vi "Update Support Build Specs and Build.vi"(7 "support build specs":T1, 8 "error in":errorcluster, 9 "CD support lvproj name":string, 10 "CD name":string, 11 "custom device path":path) -> (0 "error out":errorcluster, 3 "custom device path out":path)   [LabVIEW 2020, in "Template Tool.lvlib"]
uses:
  Template Tool.lvlib
  Project Build Specs.ctl
  <vilib>/AppBuilder/AB_API/PPL/NI_AB_API_PPL.lvclass
  <vilib>/AppBuilder/AB_API/SDIST/NI_AB_API_SDIST.lvclass
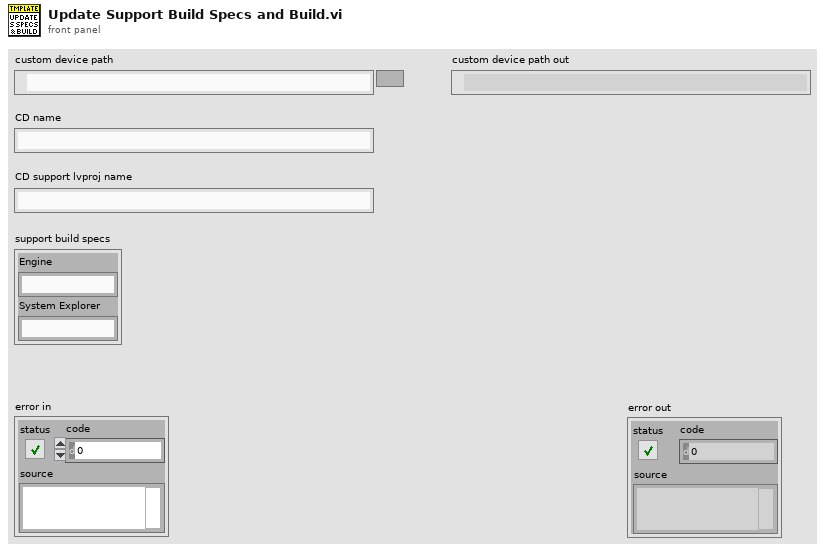
[diagram p1: front panel]
types:
  T1 = typedef "Template Tool.lvlib/Project Build Specs.ctl" = cluster{"Engine":string, "System Explorer":string}
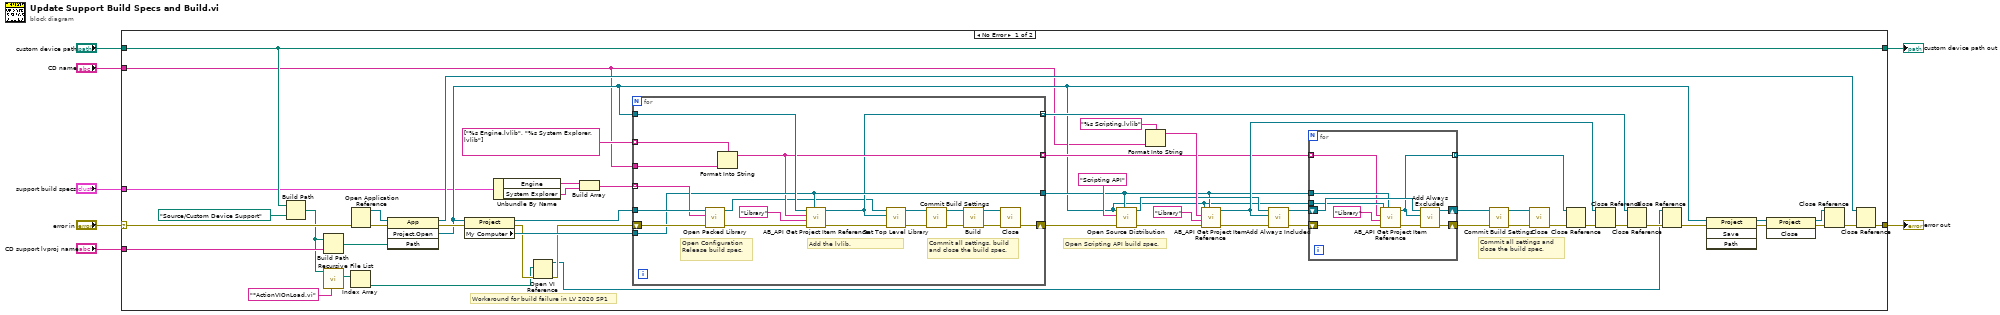
[diagram p0: block diagram]
diagram:
  n1 = case shown="No Error" "error in" {
    selector: "error in" -> [w61 w94]
    tunnel: "custom device path" -> [w53 w93]
    tunnel: [w54 w94] -> w7
    tunnel: [w53 w93] -> w4
    tunnel: "CD support lvproj name" -> [w22 _]
    tunnel: "CD name" -> [w21 _]
    tunnel: "support build specs" -> [w11 _]
    frame No Error {
      # "Workaround for build failure in LV 2020 SP1"
      # "Commit all settings and close the build spec."
      # "Open Scripting API build spec."
      n2 = Build Path(base path=w53, name or relative path=path "Source/Custom Device Support") -> (appended path=w19:path)
      n3 = Build Path(base path=w19, name or relative path=w22) -> (appended path=w20:path)
      n4 = call <vilib>:"Recursive File List.vi"("pattern"="*ActionVIOnLoad.vi", "Folder Path"=w19) -> ("All Files in Dir"=w16:path[])  [unwired: 5 in, 4 out]
      n5 = Index Array(array=w16) -> (element=w15:path)  [unwired: 1 in]
      n6 = Open Application Reference(8:w61) -> (0:w60:errorcluster, 3:w59:refnum<vi>)  [unwired: 3 in]
      n7 = invoke class="App" method="Project.Open"(reference=w59, error in=w60, "Path"=w20) -> (reference out=w52:refnum<vi>, error out=w58:errorcluster, "Project:Open"=w26:refnum<vi>)  [unwired: 1 in, 1 out]
      n8 = property class="Project"(reference=w26, error in=w58) -> (reference out=w45:refnum<vi>, error out=w17:errorcluster, "My Computer"=w44:refnum<vi>)
      n9 = Unbundle By Name(w11) -> ("Engine"=w10:string, "System Explorer"=w9:string)
      n10 = Open VI Reference(vi path=w15, error in (no error)=w17) -> (vi reference=w12:refnum<vi>, error out=w14:errorcluster)  [unwired: 4 in]
      n11 = Build Array(w10, w9) -> (w8:string[])
      n12 = for {
        tunnel: w26 -> [w89]
        tunnel: w45 -> [w87]
        tunnel: w44 -> [w84]
        tunnel: [w82] -> w36 mode=indexing
        shift-right: [w88] -> w48
        shift-left: w14 -> [w90]
        tunnel: w8 -> [w86] mode=indexing
        tunnel: string[] ["%s Engine.lvlib", "%s System Explorer.lvlib"] -> [w85] mode=indexing
        tunnel: [w84] -> w29
        tunnel: [w83] -> w28 mode=indexing
        tunnel: w21 -> [w77]
        # "Commit all settings, build and close the build spec."
        # "Add the lvlib."
        # "Open Configuration Release build spec."
        n13 = call <vilib>:"Open Packed Library.vi"("error in (no error)"=w90, "Build specification name"=w86, "Project Refnum"=w87) -> ("error out"=w91:errorcluster, "PPL out"=w81:refnum<class "NI_AB_API_PPL.lvclass">)  [unwired: 7 in]
        n14 = Format Into String(format string=w85, w77) -> (resulting string=w83:string)  [unwired: 2 in, 1 out]
        n15 = call <vilib>:"AB_API Get Project Item Reference.vi"("TargetItem Refnum"=w84, "error in (no error)"=w91, "Type"="Library", "Name"=w83, "Project Refnum"=w89) -> ("error out"=w80:errorcluster, "ProjectItem Refnum"=w82:refnum<vi>)  [unwired: 4 in, 1 out]
        n16 = call-dynamic "Set Top Level Library.vi"("error in (no error)"=w80, "ProjectItem Refnum"=w82, "PPL in"=w81) -> ("error out"=w78:errorcluster, "PPL out"=w79:refnum<class "NI_AB_API_PPL.lvclass">)  [unwired: 7 in]
        n17 = call-dynamic "Commit Build Settings.vi"("error in (no error)"=w78, "PPL in"=w79) -> ("error out"=w76:errorcluster, "PPL out"=w74:refnum<class "NI_AB_API_PPL.lvclass">)  [unwired: 8 in]
        n18 = call-dynamic "Build.vi"("error in (no error)"=w76, "PPL in"=w74) -> ("error out"=w75:errorcluster, "PPL out"=w73:refnum<class "NI_AB_API_PPL.lvclass">)  [unwired: 6 in, 2 out]
        n19 = call-dynamic "Close.vi"("error in (no error)"=w75, "DLL in"=w73) -> ("error out"=w88:errorcluster)  [unwired: 9 in]
      }
      n20 = call <vilib>:"Open Source Distribution.vi"("TargetItem Refnum"=w29, "error in (no error)"=w48, "Build specification name"="Scripting API", "Project Refnum"=w26) -> ("error out"=w50:errorcluster, "SDIST out"=w34:refnum<class "NI_AB_API_SDIST.lvclass">)  [unwired: 6 in]
      n21 = Format Into String(format string="%s Scripting.lvlib", w21) -> (resulting string=w39:string)  [unwired: 2 in, 1 out]
      n22 = call <vilib>:"AB_API Get Project Item Reference.vi"("TargetItem Refnum"=w29, "error in (no error)"=w50, "Type"="Library", "Name"=w39, "Project Refnum"=w26) -> ("error out"=w37:errorcluster, "ProjectItem Refnum"=w35:refnum<vi>)  [unwired: 4 in, 1 out]
      n23 = call-dynamic "Add Always Included.vi"("error in (no error)"=w37, "ProjectItem Refnum"=w35, "SDIST in"=w34) -> ("error out"=w33:errorcluster, "SDIST out"=w31:refnum<class "NI_AB_API_SDIST.lvclass">)  [unwired: 7 in]
      n24 = for {
        shift-right: [w72] -> w32
        shift-left: w33 -> [w65]
        shift-right: [w71] -> w30
        shift-left: w31 -> [w68]
        tunnel: w26 -> [w67]
        tunnel: w29 -> [w66]
        tunnel: w28 -> [w64] mode=indexing
        tunnel: [w63] -> w27 mode=indexing
        n25 = call <vilib>:"AB_API Get Project Item Reference.vi"("TargetItem Refnum"=w66, "error in (no error)"=w65, "Type"="Library", "Name"=w64, "Project Refnum"=w67) -> ("error out"=w69:errorcluster, "ProjectItem Refnum"=w63:refnum<vi>)  [unwired: 4 in, 1 out]
        n26 = call-dynamic "Add Always Excluded.vi"("error in (no error)"=w69, "ProjectItem Refnum"=w63, "SDIST in"=w68) -> ("error out"=w72:errorcluster, "SDIST out"=w71:refnum<class "NI_AB_API_SDIST.lvclass">)  [unwired: 7 in]
      }
      n27 = call-dynamic "Commit Build Settings.vi"("error in (no error)"=w32, "SDIST in"=w30) -> ("error out"=w46:errorcluster, "SDIST out"=w47:refnum<class "NI_AB_API_SDIST.lvclass">)  [unwired: 8 in]
      n28 = call-dynamic "Close.vi"("error in (no error)"=w46, "SDIST in"=w47) -> ("error out"=w43:errorcluster)  [unwired: 9 in]
      n29 = Close Reference(reference=w27, error in (no error)=w43) -> (error out=w42:errorcluster)
      n30 = Close Reference(reference=w35, error in (no error)=w42) -> (error out=w41:errorcluster)
      n31 = Close Reference(reference=w36, error in (no error)=w41) -> (error out=w25:errorcluster)
      n32 = Close Reference(reference=w12, error in (no error)=w25) -> (error out=w13:errorcluster)
      n33 = invoke class="Project" method="Save"(reference=w26, error in=w13) -> (reference out=w24:refnum<vi>, error out=w23:errorcluster)  [unwired: 2 in, 2 out]
      n34 = invoke class="Project" method="Close"(reference=w24, error in=w23) -> (reference out=w55:refnum<vi>, error out=w56:errorcluster)  [unwired: 1 in, 1 out]
      n35 = Close Reference(reference=w55, error in (no error)=w56) -> (error out=w57:errorcluster)
      n36 = Close Reference(reference=w52, error in (no error)=w57) -> (error out=w54:errorcluster)
    }
    frame Error {
    }
  }
  "error out" <- w7
  "custom device path out" <- w4
